vi "移位寄存器（滑动平均）.vi"() -> ()   [LabVIEW 2017]
uses:
  <vilib>/Analysis/baseanly.llb/Mean (DBL).vi
  <vilib>/Analysis/NI_AALBase.lvlib
panel:
  out "波形图表":cluster{"number: 0 to 1":dbl, "mean":dbl}(graph)
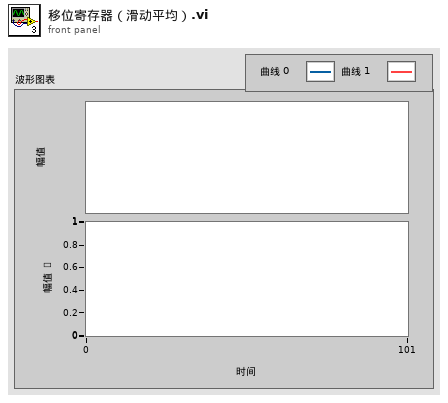
[diagram p1: front panel]
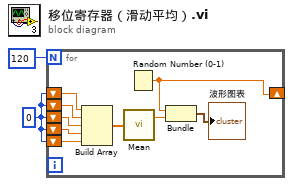
[diagram p0: block diagram]
diagram:
  w2 = 0
  n1 = for {
    N: 120 -> [_]
    shift-right: [w6] -> _
    shift-left: w2 -> [w11]
    shift-left: w2 -> [w10]
    shift-left: w2 -> [w9]
    shift-left: w2 -> [w8]
    shift-left: w2 -> [w7]
    n2 = Build Array(w11, w10, w9, w8, w7) -> (w4:dbl[])
    n3 = call-poly <vilib>:"Mean.vi"("X"=w4) -> ("mean"=w3:dbl)  [unwired: 1 out]
    n4 = Random Number (0-1)() -> (number: 0 to 1=w6:dbl)
    n5 = Bundle("number: 0 to 1"=w6, "mean"=w3) -> (→"波形图表":cluster{"number: 0 to 1":dbl, "mean":dbl})  [unwired: 1 in]
  }
